vi "FG.vi"(2 "FG Action":T1, 3 "HB in":bool) -> (1 "HB out":bool)   [LabVIEW 2009]
uses:
  cRIO/Functional Global Variables/Actions for FG's.ctl
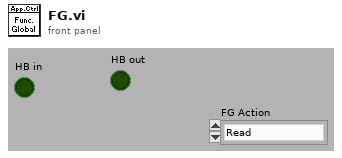
[diagram p1: front panel]
types:
  T1 = typedef "Actions for FG's.ctl" = enum16{"Read", "Write"}
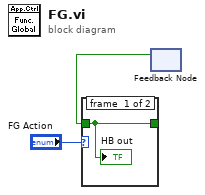
[diagram p0: block diagram]
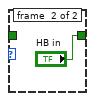
[diagram p2: hidden frame]
diagram:
  n1 = feedback #1() -> (w1:bool)  [unwired: 1 in]
  n2 = case shown="\"Write\"" "FG Action" {
    tunnel: [w4 "HB in"] -> w2
    tunnel: w1 -> [w4 _]
    frame #0 {
      "HB out" <- w4
    }
    frame #1 {
    }
  }
